vi "Arduino Pro Mini.vi"() -> (0 "Generic Device":T1={"DI Channels"=[], "DO Channels"=[], "AI"=[], "AO"=[], "PWM"=[], "QE"=[], "UART"=[], "I2C 2"=[], "SPI"=[], "CAN"=[], "AI Ref (V)"=0.0, "Firmware Program Interfaces"=[], "Firmware Versions"=[], "Name"="Arduino Pro Mini", "AO Resolution (Bits)"=0, "AO Ref (V)"=0.0})   [LabVIEW 2011, in "LVH-LINX.lvlib"]
uses:
  LVH-LINX.lvlib
  Generic Device.ctl
  Firmware Version.ctl
  Device/Type Defs/Firmware Interface.ctl
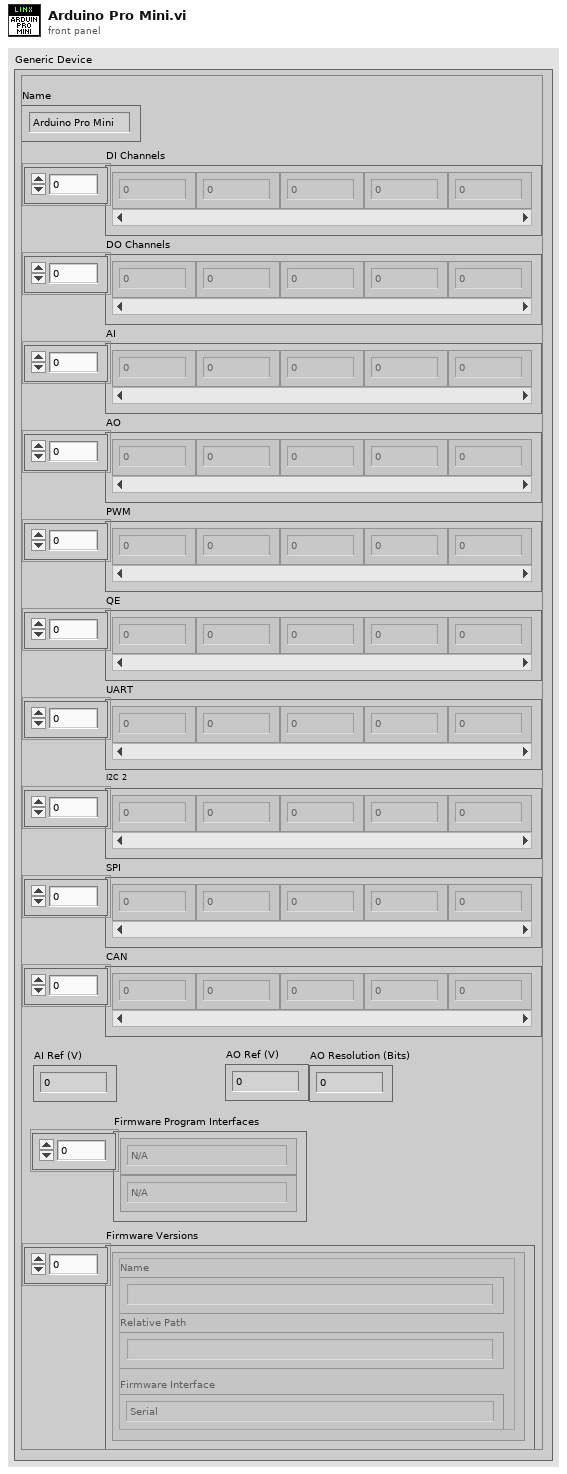
[diagram p1: front panel]
types:
  T1 = typedef "LVH-LINX.lvlib/Generic Device.ctl" = cluster{"DI Channels":u8[], "DO Channels":u8[], "AI":u8[], "AO":u8[], "PWM":u8[], "QE":u8[], "UART":u8[], "I2C 2":u8[], "SPI":u8[], "CAN":u8[], "AI Ref (V)":dbl, "Firmware Program Interfaces":enum16{"N/A", "Serial / USB", "USB", "TCP"}[], "Firmware Versions":T2[], "Name":string, "AO Resolution (Bits)":u8, "AO Ref (V)":dbl}
  T2 = typedef "LVH-LINX.lvlib/Firmware Version.ctl" = cluster{"Name":string, "Relative Path":string, "Firmware Interface":T3}
  T3 = typedef "LVH-LINX.lvlib/Firmware Interface.ctl" = enum32{"Serial ", "Ethernet", "WIFI"}
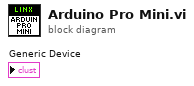
[diagram p0: block diagram]
diagram:
